vi "SLL DE Generate Time Events.vi"(8 "error in (no error)":errorcluster) -> (0 "error out":errorcluster, 3 "2 Mins":bool, 5 "Seconds":dbl)   [LabVIEW 2013]
panel:
  out "30 Mins":bool
  out "5 Mins":bool
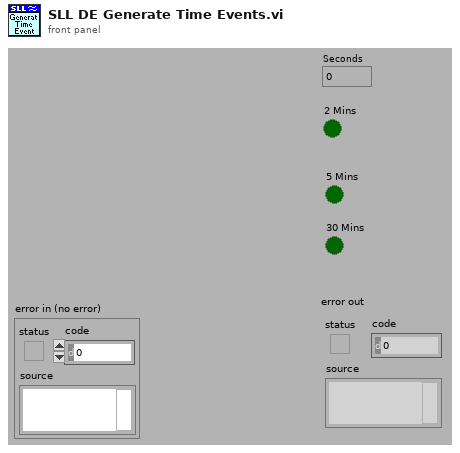
[diagram p1: front panel]
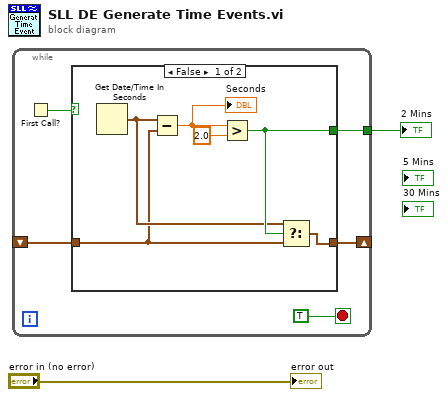
[diagram p0: block diagram]
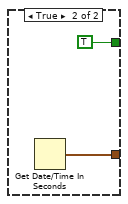
[diagram p2: hidden frame]
diagram:
  n1 = while {
    shift-right: [w5] -> _
    shift-left: _ -> [w4]
    tunnel: [w3] -> w1
    stop <- TRUE stop-if-true
    n2 = First Call?() -> (First Call?: T/F=w6:bool)
    n3 = case shown="False" w6 {
      tunnel: [w8 w15] -> w5
      tunnel: w4 -> [w9 _]
      tunnel: [w11 TRUE] -> w3
      frame False {
        n4 = Get Date/Time In Seconds() -> (seconds since 1Jan1904=w10:timestamp)
        n5 = Subtract(x=w10, y=w9) -> (x-y=w13:dbl)
        "Seconds" <- w13
        n6 = Greater?(x=w13, y=2.0) -> (0:w11:bool)
        n7 = Select(t=w10, s=w11, f=w9) -> (s? t:f=w8:timestamp)
      }
      frame True {
        n8 = Get Date/Time In Seconds() -> (seconds since 1Jan1904=w15:timestamp)
      }
    }
  }
  "2 Mins" <- w1
  "error out" <- "error in (no error)"
